vi "re_LuaVIEW Task (other 1 normal).vi"   [LabVIEW 2012]
doc: "By instantiating and running this reentrant VI, a new task execution context is created. A number of alternative copies of this VI are available that differ only in their set priority and preferred execution system. This allows selection of the priority and execution system of a new task: these properties cannot be programatically set for a VI that is not in edit mode, at least for LabVIEW versions up to 7.0."
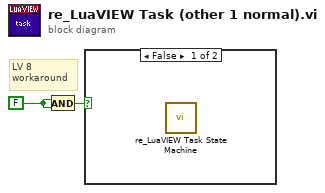
[diagram p0: block diagram]
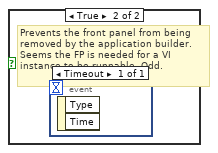
[diagram p2: hidden frame]
diagram:
  w1 = FALSE
  # "LV 8\nworkaround"
  n1 = And(x=w1, y=w1) -> (x .and. y?=w2:bool)
  n2 = case shown="False" w2 {
    frame False {
      n3 = call "re_LuaVIEW Task State Machine.vi"() -> ()  [unwired: 20 in]
    }
    frame True {
      # "Prevents the front panel from being\nremoved by the application builder.\nSeems the FP is needed for a VI\ninstance to be runnable. Odd."
      n4 = event shown="[0] Timeout" {
        selector: _ -> [_]
        dyn-events: _ -> [_]
        timeout: _ -> [_]
        event Timeout {
          n5 = event-data() -> ()  [unwired: 1 in, 2 out]
        }
      }
    }
  }
